vi "TDMS Read Example.vi"() -> ()   [LabVIEW 2016, in "LVtoITX.lvclass"]
uses:
  LVtoITX.lvclass
panel:
  in  "Read Type":enum16{"1 read", "N reads"}(ring)
  out "load time (ms)":u32
  out "Data 2":dbl[][](array[numeric]) format="%#_6p"
  in  "Waves":u16[](array[ring])
  in  "Load Multiple Waves":bool
  in  "Load Wave":bool
  in  "Load Wavenames":bool
  in  "TDMS File path":path
  in  "Stop":bool
  out "Data":dbl[](array[numeric]) format="%#_6p"
  in  "Wave":u16(ring)
  # "^^^^^^^^^^\nPush to populate the ring controls below"
  # "1 read: open file once and get all waves. Choose waves from dictionary after loading\n\nN read: open file for each wave"
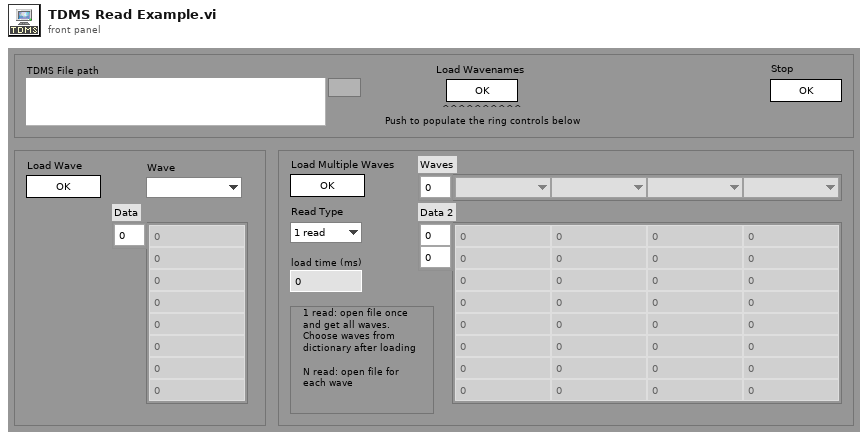
[diagram p1: front panel]
types:
  T1 = enum32{"Invalid", "Standard", "Closed", "Hidden", "Minimized", "Maximized"}
  T2 = enum32{"invalid app kind", "Development System", "Run Time System", "Student Edition", "Embedded LabVIEW", "Evaluation", "Custom"}
  T3 = cluster{"Core":cluster{"Current VI Reference":refnum<vi>, "Close Panel on Exit?":bool}, "TDMS File path":path}
  T4 = cluster{"Current VI Reference":refnum<vi>, "Close Panel on Exit?":bool}
  T5 = typedef "LVtoITX.lvclass/Dictionary--cluster.ctl" = cluster{"key":string, "value":variant}
  T6 = typedef "Dictionary Object RefNum__ogtk.ctl" = refnum<k1>
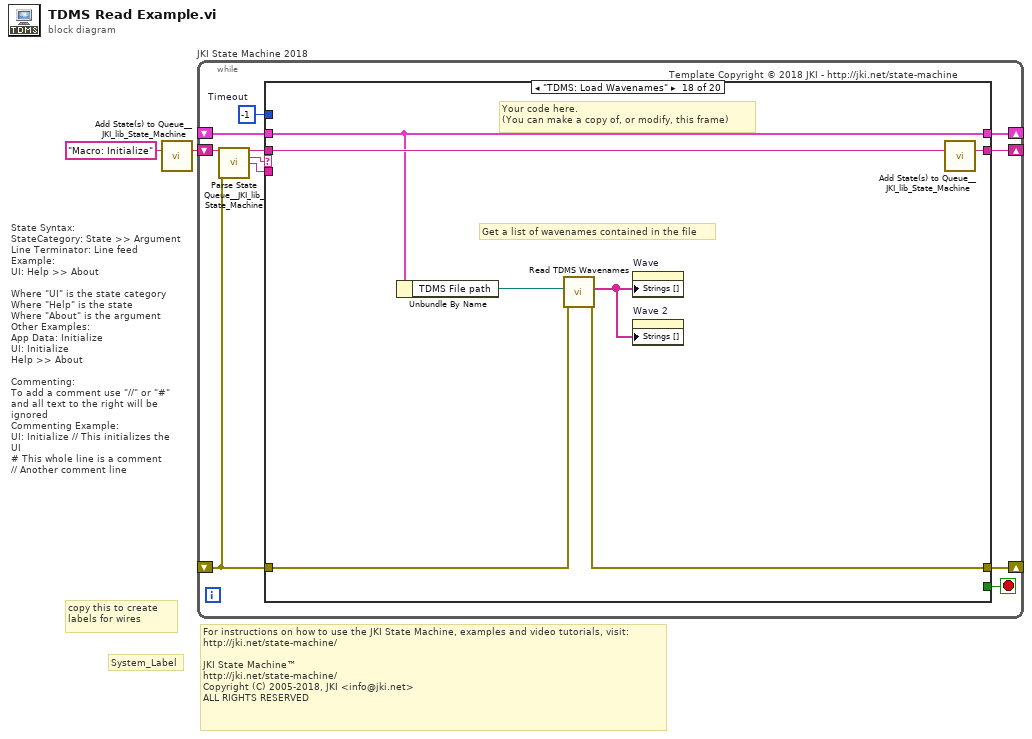
[diagram p0: block diagram]
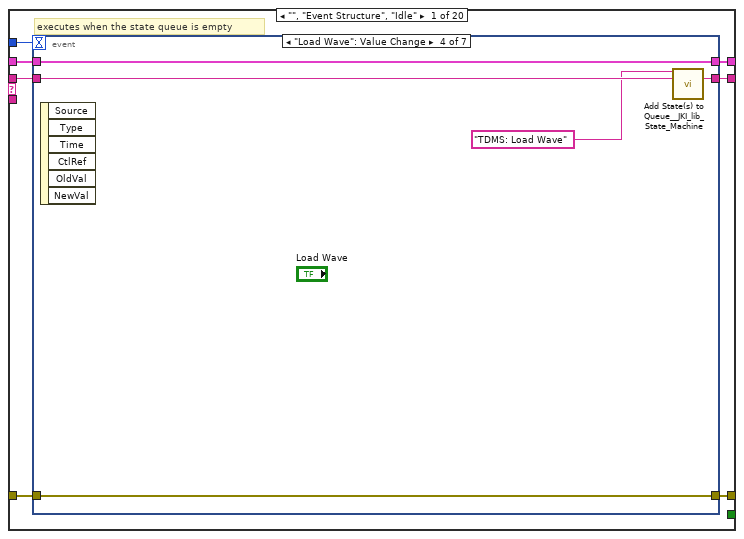
[diagram p2: hidden frame]
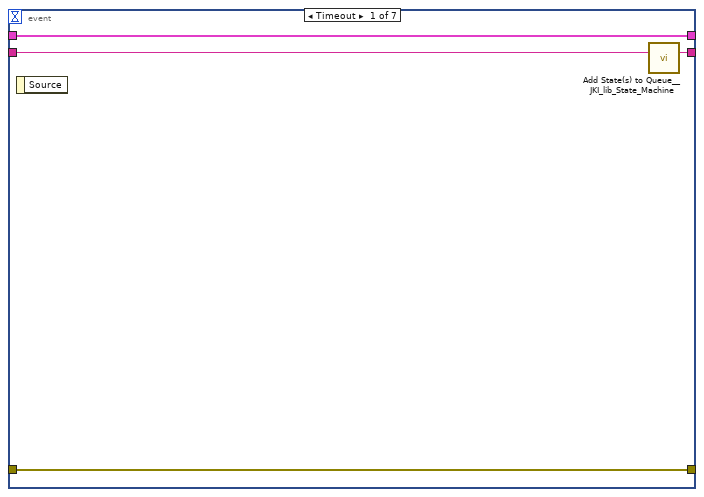
[diagram p3: hidden frame]
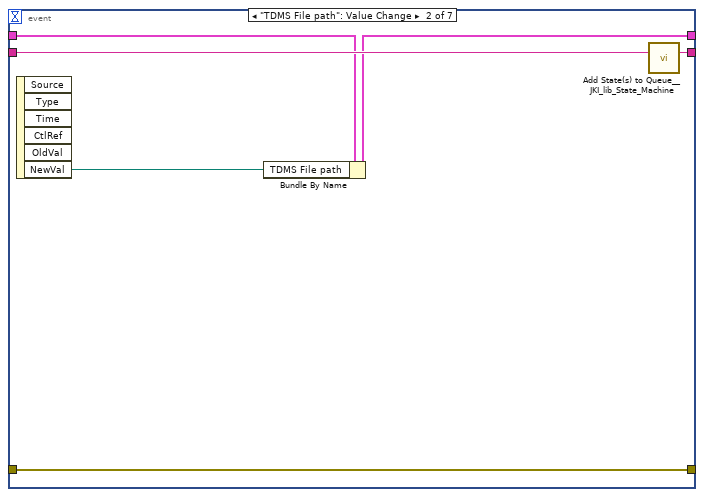
[diagram p4: hidden frame]
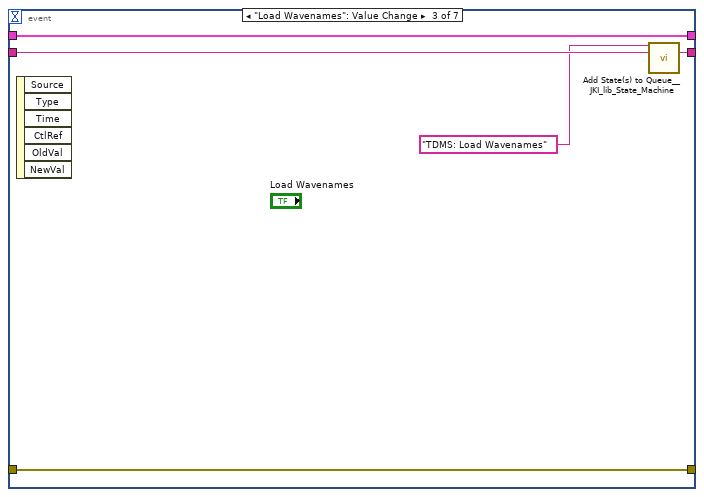
[diagram p5: hidden frame]
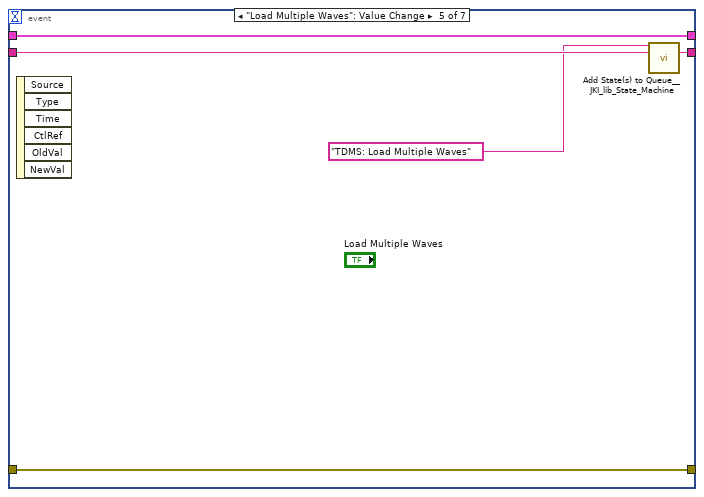
[diagram p6: hidden frame]
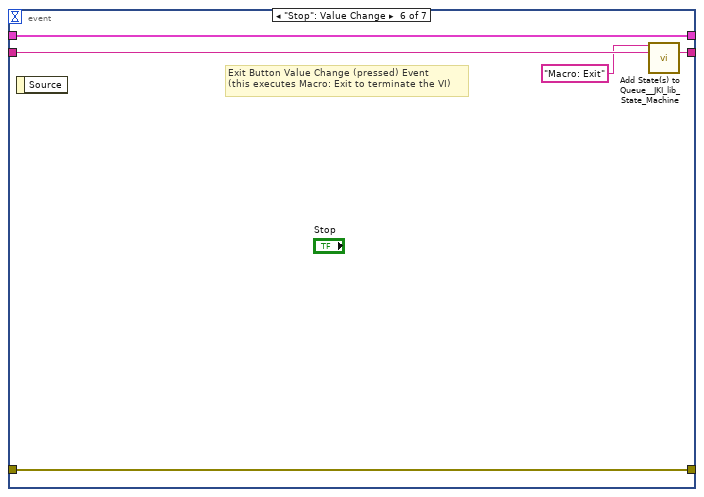
[diagram p7: hidden frame]
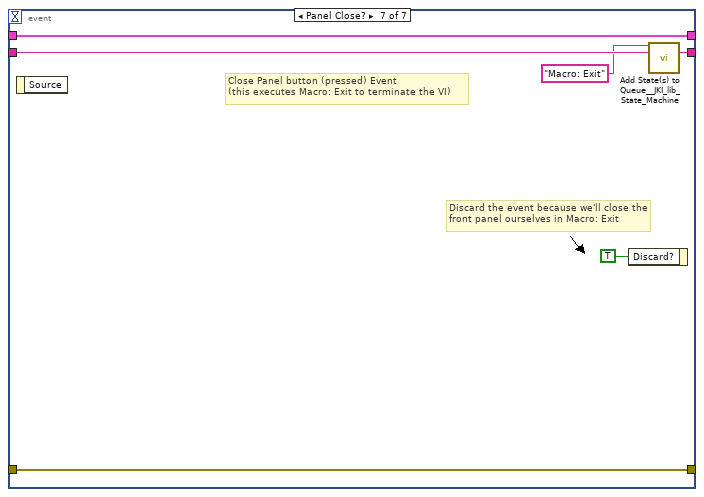
[diagram p8: hidden frame]
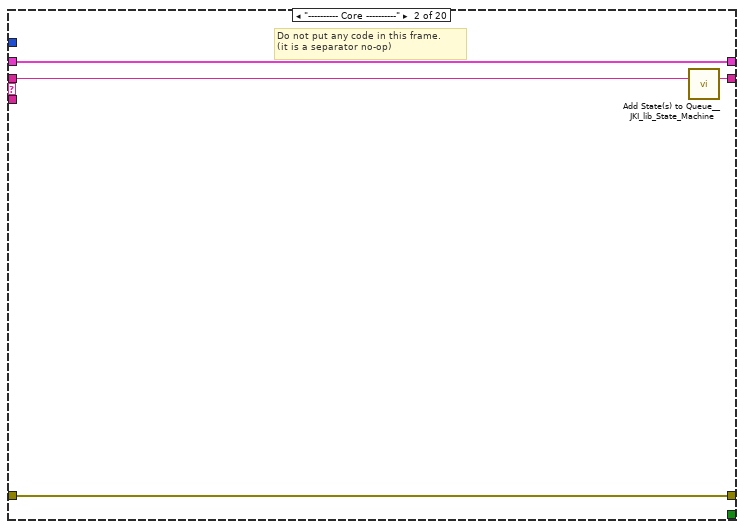
[diagram p9: hidden frame]
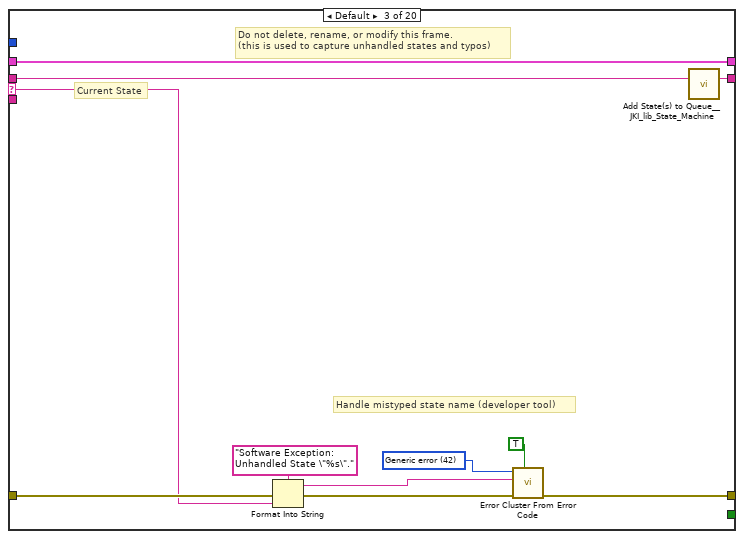
[diagram p10: hidden frame]
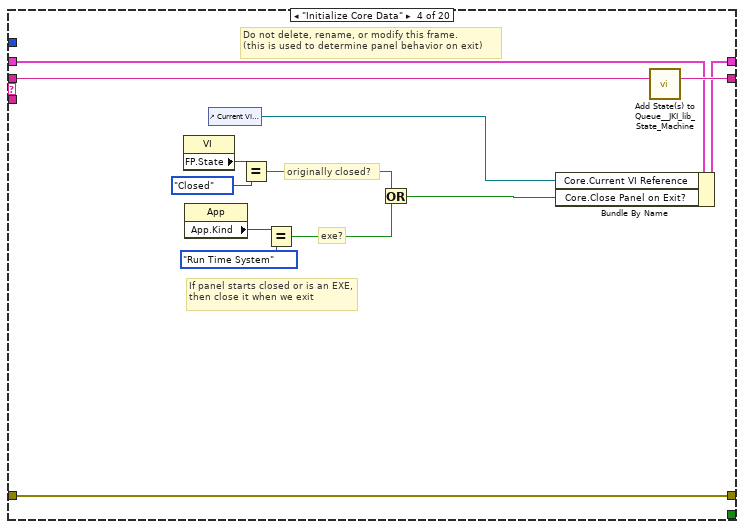
[diagram p11: hidden frame]
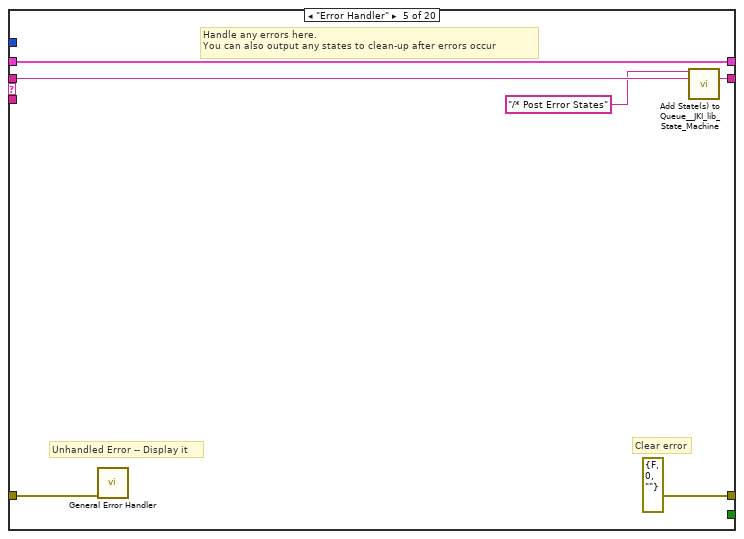
[diagram p12: hidden frame]
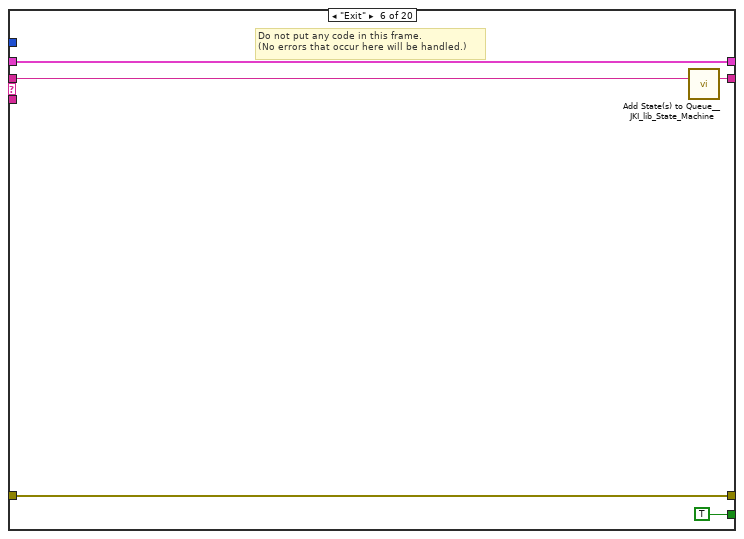
[diagram p13: hidden frame]
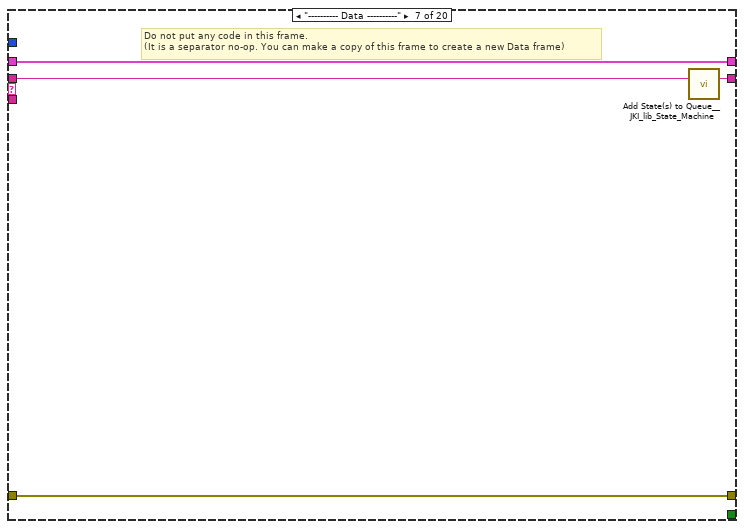
[diagram p14: hidden frame]
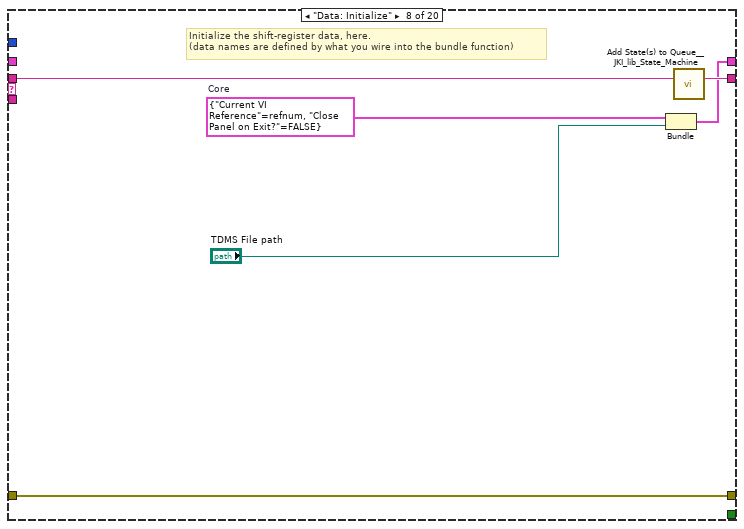
[diagram p15: hidden frame]
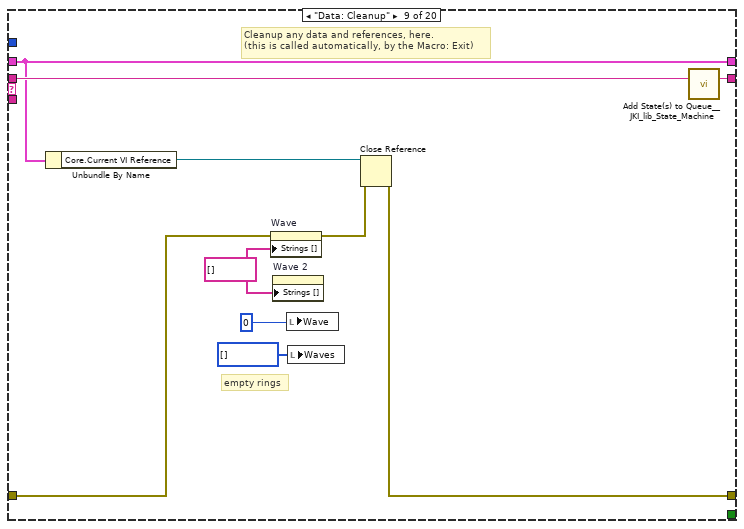
[diagram p16: hidden frame]
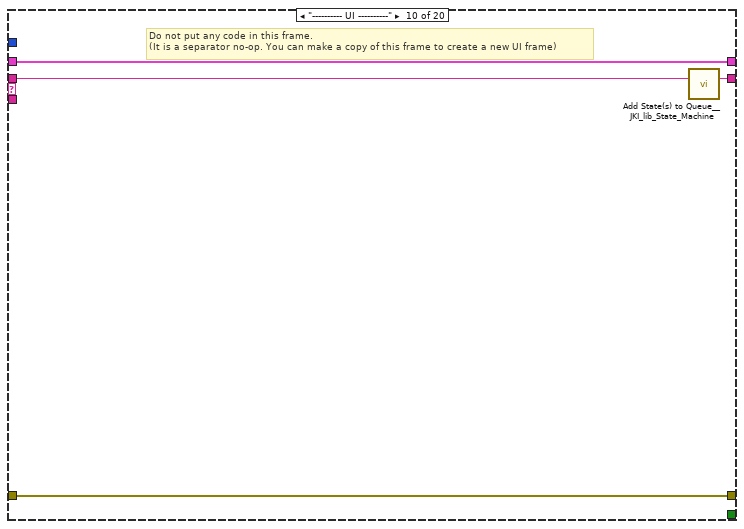
[diagram p17: hidden frame]
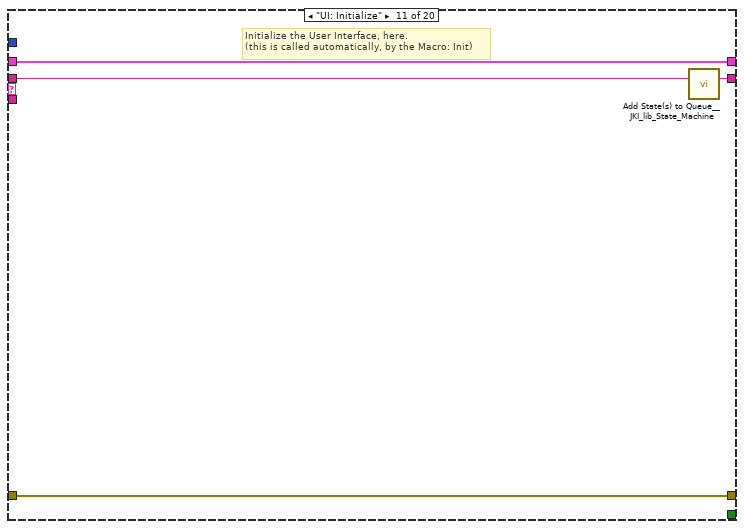
[diagram p18: hidden frame]
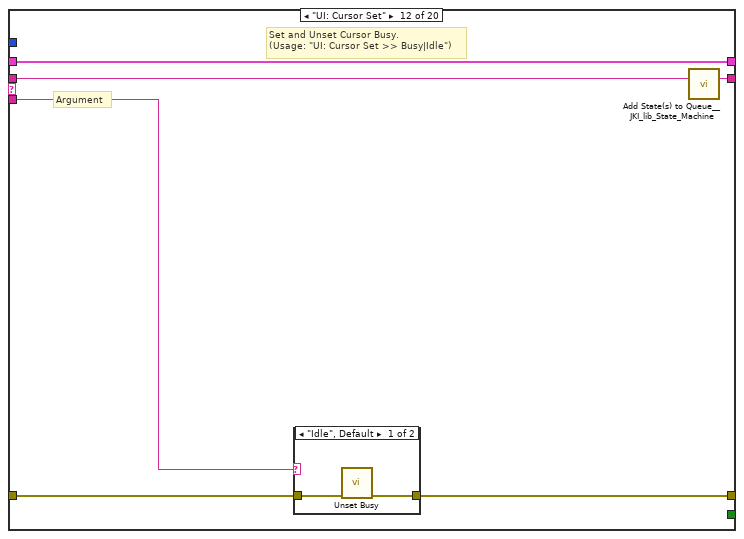
[diagram p19: hidden frame]
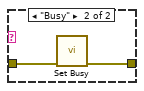
[diagram p20: hidden frame]
diagram:
  # "For instructions on how to use the JKI State Machine, examples and video tutorials, visit:\nhttp://jki.net/state-machine/\n\nJKI State Machine™\nhttp://jki.net/state-machine/\nCopyright (C) 2005-2018, JKI <info@jki.net>\nALL RIGHTS RESERVED"
  # "State Syntax:\nStateCategory: State >> Argument\nLine Terminator: Line feed\nExample:\nUI: Help >> About\n\nWhere \"UI\" is the state category\nWhere \"Help\" is the state\nWhere \"About\" is the argument\nOther Examples:\nApp Data: Initialize\nUI: Initialize\nHelp >> About\n\nCommenting:\nTo add a comment use \"//\" or \"#\" and all text to the right will be ignored\nCommenting Example:\nUI: Initialize // This initializes the UI\n# This whole line is a comment\n// Another comment line"
  # "copy this to create labels for wires"
  # "System_Label"
  n1 = call <vilib>:"Add State(s) to Queue__JKI_lib_State_Machine.vi"("State(s) in (\"\")"="Macro: Initialize") -> ("States Out"=w2:string)  [unwired: 14 in]
  n2 = while "JKI State Machine 2018" {
    shift-right: [w6] -> _
    shift-left: _ -> [w5]
    shift-right: [w9] -> _
    shift-left: _ -> [w3]
    shift-right: [w8] -> _
    shift-left: w2 -> [w10]
    stop <- w7 stop-if-true
    w4 = -1  # Timeout
    # "Template Copyright © 2018 JKI - http://jki.net/state-machine"
    n3 = call <vilib>:"Parse State Queue__JKI_lib_State_Machine.vi"("State Queue"=w10, "Error In (no error)"=w3) -> ("Remaining States"=w12:string, "Current State"=w13:string, "Arguments"=w11:string)  [unwired: 11 in]
    n4 = case shown="\"TDMS: Load Wavenames\"" w13 {
      selector: w13 -> [_ _ w61 _ _ _ _ _ _ _ _ _ _ _ _ _ _ _ _ _]
      tunnel: w12 -> [w20 w60 w65 w84 w90 w95 w99 w105 w115 w119 w123 w129 w140 w209 w214 w224 w228 w235 w245 w261]
      tunnel: w11 -> [_ _ _ _ _ _ _ _ _ _ _ w124 w134 _ _ _ _ _ _ _]
      tunnel: w5 -> [w18 w57 w63 w77 w87 w93 w96 _ w111 w116 w121 w127 w136 w206 w211 w221 w225 w230 w237 w259]
      tunnel: [w17 w58 w67 w81 errorcluster {"status"=FALSE, "code"=0, "source"=""} ("error out") w92 w97 w102 w112 w117 w120 w125 w137 w207 w212 w222 w226 w232 w240 w253] -> w9
      tunnel: w3 -> [w16 w58 w66 w81 w86 w92 w97 w102 w110 w117 w120 w126 w138 w207 w212 w222 w226 w233 w241 w254]
      tunnel: [w19 w59 w64 w83 w89 w94 w98 w104 w114 w118 w122 w128 w139 w208 w213 w223 w227 w234 w244 w260] -> w8
      tunnel: [_ _ _ _ _ TRUE _ _ _ _ _ _ _ _ _ _ _ _ _ _] -> w7
      tunnel: [w15 w57 w63 w82 w87 w93 w96 w103 w111 w116 w121 w127 w136 w206 w211 w221 w225 w230 w237 w259] -> w6
      tunnel: w4 -> [w14 _ _ _ _ _ _ _ _ _ _ _ _ _ _ _ _ _ _ _]
      frame "", "Event Structure", "Idle" {
        # "executes when the state queue is empty"
        n5 = event shown="[3] \"Load Wave\": Value Change" {
          selector: _ -> [_ _ _ _ _ _ _]
          dyn-events: _ -> [_ _ _ _ _ _ _]
          timeout: w14 -> [_ _ _ _ _ _ _]
          tunnel: w20 -> [w24 w30 w35 w40 w45 w50 w56]
          tunnel: [w23 w29 w34 w39 w44 w49 w55] -> w19
          tunnel: w18 -> [w21 w26 w32 w37 w42 w47 w53]
          tunnel: [w22 w28 w33 w38 w43 w48 w54] -> w17
          tunnel: w16 -> [w22 w28 w33 w38 w43 w48 w54]
          tunnel: [w21 w25 w32 w37 w42 w47 w53] -> w15
          event Timeout {
            n6 = event-data() -> ()  [unwired: 1 in, 1 out]
            n7 = call <vilib>:"Add State(s) to Queue__JKI_lib_State_Machine.vi"("State(s) in (\"\")"=w24) -> ("States Out"=w23:string)  [unwired: 14 in]
          }
          event "TDMS File path": Value Change {
            n8 = event-data() -> ("NewVal"=w27:path)  [unwired: 1 in, 5 out]
            n9 = Bundle By Name(cluster=w26, "TDMS File path"=w27) -> (w25:T3)
            n10 = call <vilib>:"Add State(s) to Queue__JKI_lib_State_Machine.vi"("State(s) in (\"\")"=w30) -> ("States Out"=w29:string)  [unwired: 14 in]
          }
          event "Load Wavenames": Value Change {
            n11 = event-data() -> ()  [unwired: 1 in, 6 out]
            n12 = call <vilib>:"Add State(s) to Queue__JKI_lib_State_Machine.vi"("State(s) in Front (\"\")"="TDMS: Load Wavenames" ("State(s) in Front (\"\")"), "State(s) in (\"\")"=w35) -> ("States Out"=w34:string)  [unwired: 13 in]
          }
          event "Load Wave": Value Change {
            n13 = event-data() -> ()  [unwired: 1 in, 6 out]
            n14 = call <vilib>:"Add State(s) to Queue__JKI_lib_State_Machine.vi"("State(s) in Front (\"\")"="TDMS: Load Wave" ("State(s) in Front (\"\")"), "State(s) in (\"\")"=w40) -> ("States Out"=w39:string)  [unwired: 13 in]
          }
          event "Load Multiple Waves": Value Change {
            n15 = event-data() -> ()  [unwired: 1 in, 6 out]
            n16 = call <vilib>:"Add State(s) to Queue__JKI_lib_State_Machine.vi"("State(s) in Front (\"\")"="TDMS: Load Multiple Waves" ("State(s) in Front (\"\")"), "State(s) in (\"\")"=w45) -> ("States Out"=w44:string)  [unwired: 13 in]
          }
          event "Stop": Value Change {
            # "Exit Button Value Change (pressed) Event\n(this executes Macro: Exit to terminate the VI)"
            n17 = event-data() -> ()  [unwired: 1 in, 1 out]
            n18 = call <vilib>:"Add State(s) to Queue__JKI_lib_State_Machine.vi"("State(s) in Front (\"\")"="Macro: Exit", "State(s) in (\"\")"=w50) -> ("States Out"=w49:string)  [unwired: 13 in]
          }
          event Panel Close? {
            # "Discard the event because we'll close the front panel ourselves in Macro: Exit"
            # "Close Panel button (pressed) Event\n(this executes Macro: Exit to terminate the VI)"
            n19 = event-data() -> ()  [unwired: 1 in, 1 out]
            n20 = event-data("Discard?"=TRUE) -> ()  [unwired: 1 in, 1 out]
            n21 = call <vilib>:"Add State(s) to Queue__JKI_lib_State_Machine.vi"("State(s) in Front (\"\")"="Macro: Exit", "State(s) in (\"\")"=w56) -> ("States Out"=w55:string)  [unwired: 13 in]
          }
        }
      }
      frame "---------- Core ----------" {
        # "Do not put any code in this frame.\n(it is a separator no-op)"
        n22 = call <vilib>:"Add State(s) to Queue__JKI_lib_State_Machine.vi"("State(s) in (\"\")"=w60) -> ("States Out"=w59:string)  [unwired: 14 in]
      }
      frame Default {
        w70 = 42 items=["No error", "Argument error", "Memory is full", "Out of zone", "End of file", "File already open", "Generic file I/O error", "File not found", "File permission error", "Disk is full", "Duplicate path", "Too many files open", "System feature not enabled", "Resource file not found", "Cannot add resource", "Resource not found", "Image not found", "Image memory error", "Pen does not exist", "Config type invalid", "Config token not found", "Config parse error", "Config memory error", "Bad external code format", "Bad external code offset", "External code not present", "Null window", "Destroy window error", "Null menu", "Print aborted", "Bad print record", "Print driver error", "Windows error during printing", "Memory error during printing", "Print dialog error", "Generic print error", "Invalid device refnum", "Device not found", "Device parameter error", "Device unit error", "Cannot open device", "Device call aborted", "Generic error", "Cancelled by user", "Object ID too low", "Object ID too high", "Object not in heap", "Unknown heap", "Unknown object (invalid DefProc)", "Unknown object (DefProc not in table)", "Message out of range", "Invalid (null) method", "Unknown message", "Manager call not supported", "Bad address", "Network operation in progress", "Network operation timed out", "Connection is busy", "Network attribute not supported", "Network error", "Address in use", "System out of memory", "Connection aborted", "Connection refused", "Not connected", "Already connected", "Connection closed", "Initialization error (interapplication manager)", "Bad occurrence", "Wait on unbound occurrence handler", "Occurrence queue overflow", "Datalog type conflict", "Unused", "Unrecognized type (interapplication manager)", "Memory corrupt", "Failed to make temporary DLL", "Old CIN version", "Drag socket not found", "Failed to load drop-object", "Failed to register OLE object", "Failed to release OLE object", "Format specifier type mismatch", "Unknown format specifier", "Too few format specifiers", "Too many format specifiers", "Scan failed", "Newer CIN version", "Error converting to variant", "Runtime menu error", "Password tampered", "Variant attribute not found", "Incompatible variant data type", "Event data is not available", "Event Store is not present", "Occurrence is not found", "Event Queue is not created", "Event info is not available", "Refnum passed is NULL", "Error retrieving Class GUID", "Error retrieving CoClass GUID", "Error retrieving TypeLib GUID.", "Bad built application magic bytes.", "Specific driver is different from the specific driver associated with the Logical Name.", "There is no session opened to the class driver.", "Max Error", "MAX - Error with config objects", "MAX - Error loading configuration", "MAX - Group not supported"]
        # "Current State"
        # "Do not delete, rename, or modify this frame.\n(this is used to capture unhandled states and typos)"
        # "Handle mistyped state name (developer tool)"
        n23 = Format Into String(format string="Software Exception: Unhandled State \"%s\"." ("message"), error in=w66, w61) -> (resulting string=w69:string, error out=w68:errorcluster)  [unwired: 1 in]
        n24 = call <vilib>:"Error Cluster From Error Code.vi"("show call chain? (False)"=TRUE, "error in (no error)"=w68, "error message (\"\")"=w69, "error code (0)"=w70) -> ("error out"=w67:errorcluster)  [unwired: 5 in]
        n25 = call <vilib>:"Add State(s) to Queue__JKI_lib_State_Machine.vi"("State(s) in (\"\")"=w65) -> ("States Out"=w64:string)  [unwired: 14 in]
      }
      frame "Initialize Core Data" {
        # "Do not delete, rename, or modify this frame.\n(this is used to determine panel behavior on exit)"
        # "originally closed?"
        # "exe?"
        # "If panel starts closed or is an EXE, then close it when we exit"
        n26 = property class="VI"() -> ("FP.State"=w74:T1)  [unwired: 2 in, 2 out]
        n27 = property class="App"() -> ("App.Kind"=w80:T2)  [unwired: 2 in, 2 out]
        n28 = control-ref of="Current VI Reference"() -> (w75:refnum<vi>)
        n29 = Equal?(x=w74, y=T1."Closed" ("Front Panel Window:State")) -> (x = y?=w72:bool)
        n30 = Equal?(x=w80, y=T2."Run Time System" ("Application:Kind")) -> (x = y?=w78:bool)
        n31 = Or(x=w72, y=w78) -> (x .or. y?=w76:bool)
        n32 = Bundle By Name(cluster=w77, "Core.Current VI Reference"=w75, "Core.Close Panel on Exit?"=w76) -> (w82:T3)
        n33 = call <vilib>:"Add State(s) to Queue__JKI_lib_State_Machine.vi"("State(s) in (\"\")"=w84) -> ("States Out"=w83:string)  [unwired: 14 in]
      }
      frame "Error Handler" {
        # "Unhandled Error -- Display it"
        # "Handle any errors here.\nYou can also output any states to clean-up after errors occur"
        # "Clear error"
        n34 = call <vilib>:"General Error Handler.vi"("error in (no error)"=w86) -> ()  [unwired: 10 in, 5 out]
        n35 = call <vilib>:"Add State(s) to Queue__JKI_lib_State_Machine.vi"("State(s) in Front (\"\")"="/* Post Error States", "State(s) in (\"\")"=w90) -> ("States Out"=w89:string)  [unwired: 13 in]
      }
      frame "Exit" {
        # "Do not put any code in this frame.\n(No errors that occur here will be handled.)"
        n36 = call <vilib>:"Add State(s) to Queue__JKI_lib_State_Machine.vi"("State(s) in (\"\")"=w95) -> ("States Out"=w94:string)  [unwired: 14 in]
      }
      frame "---------- Data ----------" {
        # "Do not put any code in this frame.\n(It is a separator no-op. You can make a copy of this frame to create a new Data frame)"
        n37 = call <vilib>:"Add State(s) to Queue__JKI_lib_State_Machine.vi"("State(s) in (\"\")"=w99) -> ("States Out"=w98:string)  [unwired: 14 in]
      }
      frame "Data: Initialize" {
        w101 = T4 {"Current VI Reference"=refnum, "Close Panel on Exit?"=FALSE}  # Core
        # "Initialize the shift-register data, here.\n(data names are defined by what you wire into the bundle function)"
        n38 = Bundle("Core"=w101, "TDMS File path"="TDMS File path") -> (w103:T3)  [unwired: 1 in]
        n39 = call <vilib>:"Add State(s) to Queue__JKI_lib_State_Machine.vi"("State(s) in (\"\")"=w105) -> ("States Out"=w104:string)  [unwired: 14 in]
      }
      frame "Data: Cleanup" {
        w106 = u16[] [] items=[""] ("Waves")
        w107 = string[] [] ("Strings []")
        # "empty rings"
        # "Cleanup any data and references, here.\n(this is called automatically, by the Macro: Exit)"
        n40 = Unbundle By Name(w111) -> ("Core.Current VI Reference"=w113:refnum<vi>)
        n41 = property on="Wave" class="Ring (strict)"(error in=w110, "Strings []"=w107) -> (error out=w109:errorcluster)  [unwired: 1 in, 1 out]
        n42 = property on="Wave 2" class="Ring (strict)"("Strings []"=w107) -> ()  [unwired: 2 in, 2 out]
        n43 = local write "Wave"(0) -> ()
        n44 = local write "Waves"(w106) -> ()
        n45 = Close Reference(reference=w113, error in (no error)=w109) -> (error out=w112:errorcluster)
        n46 = call <vilib>:"Add State(s) to Queue__JKI_lib_State_Machine.vi"("State(s) in (\"\")"=w115) -> ("States Out"=w114:string)  [unwired: 14 in]
      }
      frame "---------- UI ----------" {
        # "Do not put any code in this frame.\n(It is a separator no-op. You can make a copy of this frame to create a new UI frame)"
        n47 = call <vilib>:"Add State(s) to Queue__JKI_lib_State_Machine.vi"("State(s) in (\"\")"=w119) -> ("States Out"=w118:string)  [unwired: 14 in]
      }
      frame "UI: Initialize" {
        # "Initialize the User Interface, here.\n(this is called automatically, by the Macro: Init)"
        n48 = call <vilib>:"Add State(s) to Queue__JKI_lib_State_Machine.vi"("State(s) in (\"\")"=w123) -> ("States Out"=w122:string)  [unwired: 14 in]
      }
      frame "UI: Cursor Set" {
        # "Argument"
        # "Set and Unset Cursor Busy.\n(Usage: \"UI: Cursor Set >> Busy|Idle\")"
        n49 = case shown="\"Idle\", Default" w124 {
          tunnel: w126 -> [w131 w133]
          tunnel: [w130 w132] -> w125
          frame "Idle", Default {
            n50 = call <vilib>:"Unset Busy.vi"("error in (no error)"=w131) -> ("error out"=w130:errorcluster)  [unwired: 10 in]
          }
          frame "Busy" {
            n51 = call <vilib>:"Set Busy.vi"("error in (no error)"=w133) -> ("error out"=w132:errorcluster)  [unwired: 9 in, 1 out]
          }
        }
        n52 = call <vilib>:"Add State(s) to Queue__JKI_lib_State_Machine.vi"("State(s) in (\"\")"=w129) -> ("States Out"=w128:string)  [unwired: 14 in]
      }
      frame "UI: Front Panel State" {
        # "Argument"
        # "Set Front Panel Open or Closed\n(Usage: \"UI: Front Panel State >> Open|Close\")"
        n53 = Unbundle By Name(w136) -> ("Core.Current VI Reference"=w135:refnum<vi>)
        n54 = case shown="\"Minimize\", \"Minimized\"" w134 {
          tunnel: w138 -> [w146 w161 w172 w185 w198]
          tunnel: [w148 w162 w174 w187 w200] -> w137
          tunnel: w135 -> [w147 w159 w173 w186 w199]
          frame "Open", "Standard", Default {
            w141 = T1."Standard" ("State")
            n55 = property class="VI"(reference=w147, error in=w146) -> (reference out=w144:refnum<vi>, error out=w145:errorcluster, "FP.State"=w143:T1)
            n56 = Not Equal?(x=w143, y=w141) -> (x != y?=w142:bool)
            n57 = case shown="True" w142 {
              tunnel: [w152 w154] -> w148
              tunnel: w145 -> [w151 w154]
              tunnel: w144 -> [w150 _]
              tunnel: w141 -> [w149 _]
              frame True {
                n58 = invoke class="VI" method="FP.Open"(reference=w150, error in=w151, "Activate"=TRUE, "State"=w149) -> (error out=w152:errorcluster)  [unwired: 1 in, 4 out]
              }
              frame False {
              }
            }
          }
          frame "Close", "Closed" {
            n59 = property class="VI"(reference=w159, error in=w161) -> (reference out=w158:refnum<vi>, error out=w160:errorcluster, "FP.State"=w156:T1)
            n60 = Not Equal?(x=w156, y=T1."Closed" ("Front Panel Window:State")) -> (x != y?=w155:bool)
            n61 = case shown="True" w155 {
              tunnel: [w163 w166] -> w162
              tunnel: w160 -> [w163 w165]
              tunnel: w158 -> [_ w164]
              frame False {
              }
              frame True {
                n62 = invoke class="VI" method="FP.Close"(reference=w164, error in=w165) -> (error out=w166:errorcluster)  [unwired: 1 in, 2 out]
              }
            }
          }
          frame "Hidden", "Hide" {
            w167 = T1."Hidden" ("State")
            n63 = property class="VI"(reference=w173, error in=w172) -> (reference out=w170:refnum<vi>, error out=w171:errorcluster, "FP.State"=w169:T1)
            n64 = Not Equal?(x=w169, y=w167) -> (x != y?=w168:bool)
            n65 = case shown="True" w168 {
              tunnel: [w178 w179] -> w174
              tunnel: w171 -> [w177 w179]
              tunnel: w170 -> [w176 _]
              tunnel: w167 -> [w175 _]
              frame True {
                n66 = invoke class="VI" method="FP.Open"(reference=w176, error in=w177, "State"=w175) -> (error out=w178:errorcluster)  [unwired: 2 in, 4 out]
              }
              frame False {
              }
            }
          }
          frame "Minimize", "Minimized" {
            w180 = T1."Minimized" ("State")
            n67 = property class="VI"(reference=w186, error in=w185) -> (reference out=w183:refnum<vi>, error out=w184:errorcluster, "FP.State"=w182:T1)
            n68 = Not Equal?(x=w182, y=w180) -> (x != y?=w181:bool)
            n69 = case shown="True" w181 {
              tunnel: [w191 w192] -> w187
              tunnel: w184 -> [w190 w192]
              tunnel: w183 -> [w189 _]
              tunnel: w180 -> [w188 _]
              frame True {
                n70 = invoke class="VI" method="FP.Open"(reference=w189, error in=w190, "State"=w188) -> (error out=w191:errorcluster)  [unwired: 2 in, 4 out]
              }
              frame False {
              }
            }
          }
          frame "Maximize", "Maximized" {
            w193 = T1."Maximized" ("State")
            n71 = property class="VI"(reference=w199, error in=w198) -> (reference out=w196:refnum<vi>, error out=w197:errorcluster, "FP.State"=w195:T1)
            n72 = Not Equal?(x=w195, y=w193) -> (x != y?=w194:bool)
            n73 = case shown="True" w194 {
              tunnel: [w204 w205] -> w200
              tunnel: w197 -> [w203 w205]
              tunnel: w196 -> [w202 _]
              tunnel: w193 -> [w201 _]
              frame True {
                n74 = invoke class="VI" method="FP.Open"(reference=w202, error in=w203, "State"=w201) -> (error out=w204:errorcluster)  [unwired: 2 in, 4 out]
              }
              frame False {
              }
            }
          }
        }
        n75 = call <vilib>:"Add State(s) to Queue__JKI_lib_State_Machine.vi"("State(s) in (\"\")"=w140) -> ("States Out"=w139:string)  [unwired: 14 in]
      }
      frame "---------- Macro ----------" {
        # "Do not put any code in this frame.\n(It is a separator no-op. You can make a copy of this frame to create a new Macro frame)"
        n76 = call <vilib>:"Add State(s) to Queue__JKI_lib_State_Machine.vi"("State(s) in (\"\")"=w209) -> ("States Out"=w208:string)  [unwired: 14 in]
      }
      frame "Macro: Initialize" {
        w210 = "Data: Initialize\nInitialize Core Data\nUI: Initialize\nUI: Front Panel State >> Open"  # Data: Initialize Initialize Core Data UI: Initialize UI: Front Panel State >> Open
        # "Initialization Macro\n(This is called once, when the VI starts)"
        n77 = call <vilib>:"Add State(s) to Queue__JKI_lib_State_Machine.vi"("State(s) in Front (\"\")"=w210, "State(s) in (\"\")"=w214) -> ("States Out"=w213:string)  [unwired: 13 in]
      }
      frame "Macro: Exit" {
        # "Exit Macro\n(This is called once, when the VI exits)"
        n78 = Unbundle By Name(w221) -> ("Core.Close Panel on Exit?"=w220:bool)
        n79 = Select(t="UI: Front Panel State >> Close", s=w220, f="") -> (s? t:f=w217:string)
        n80 = call <vilib>:"Add State(s) to Queue__JKI_lib_State_Machine.vi"("State(s) in (\"\")"=w217, "State(s) at Back (\"\")"="Data: Cleanup\nExit") -> ("States Out"=w215:string)  [unwired: 13 in]
        n81 = call <vilib>:"Add State(s) to Queue__JKI_lib_State_Machine.vi"("State(s) in Front (\"\")"=w215, "State(s) in (\"\")"=w224) -> ("States Out"=w223:string)  [unwired: 13 in]
      }
      frame "---------- TDMS ----------" {
        # "Template Separator\n(You can make a copy of, or modify, this frame)"
        n82 = call <vilib>:"Add State(s) to Queue__JKI_lib_State_Machine.vi"("State(s) in (\"\")"=w228) -> ("States Out"=w227:string)  [unwired: 14 in]
      }
      frame "TDMS: Load Wavenames" {
        # "Get a list of wavenames contained in the file"
        # "Your code here.\n(You can make a copy of, or modify, this frame)"
        n83 = Unbundle By Name(w230) -> ("TDMS File path"=w229:path)
        n84 = call "Read TDMS Wavenames.vi"("error in (no error)"=w233, "path"=w229) -> ("error out"=w232:errorcluster, "Wavenames"=w231:string[])  [unwired: 7 in, 1 out]
        n85 = property on="Wave" class="Ring (strict)"("Strings []"=w231) -> ()  [unwired: 2 in, 2 out]
        n86 = property on="Wave 2" class="Ring (strict)"("Strings []"=w231) -> ()  [unwired: 2 in, 2 out]
        n87 = call <vilib>:"Add State(s) to Queue__JKI_lib_State_Machine.vi"("State(s) in (\"\")"=w235) -> ("States Out"=w234:string)  [unwired: 14 in]
      }
      frame "TDMS: Load Wave" {
        # "Your code here.\n(You can make a copy of, or modify, this frame)"
        n88 = Unbundle By Name(w237) -> ("TDMS File path"=w236:path)
        n89 = property on="Wave" class="Ring (strict)"() -> ("Strings []"=w243:string[])  [unwired: 2 in, 2 out]
        n90 = Index Array(array=w243, index="Wave") -> (element=w242:string)
        n91 = call "Read TDMS Wave.vi"("error in (no error)"=w241, "channel name(s) in"=w242, "path"=w236) -> ("error out"=w240:errorcluster, "data"=→"Data":dbl[])  [unwired: 6 in, 1 out]
        n92 = call <vilib>:"Add State(s) to Queue__JKI_lib_State_Machine.vi"("State(s) in (\"\")"=w245) -> ("States Out"=w244:string)  [unwired: 14 in]
      }
      frame "TDMS: Load Multiple Waves" {
        # "Template Separator\n(You can make a copy of, or modify, this frame)"
        n93 = Unbundle By Name(w259) -> ("TDMS File path"=w258:path)
        n94 = property on="Wave 2" class="Ring (strict)"() -> ("Strings []"=w256:string[])  [unwired: 2 in, 2 out]
        n95 = call <userlib>:"Tick Count (ms)__ogtk.vi"("error in (no error)"=w254) -> ("error out"=w251:errorcluster, "millisecond timer value"=w250:u32)  [unwired: 9 in]
        n96 = case shown="\"1 read\", Default" "Read Type" {
          tunnel: w258 -> [w272 w289]
          tunnel: "Waves" -> [w269 w287]
          tunnel: w256 -> [w268 w286]
          tunnel: [w266 w285] -> w255
          tunnel: [w264 w284] -> w252
          tunnel: w251 -> [w263 w288]
          frame "1 read", Default {
            n97 = call "Read TDMS.vi"("error in (no error)"=w263, "path"=w272) -> ("error out"=w267:errorcluster, "Data (Dictionary)"=w271:T5[])  [unwired: 3 in, 5 out]
            n98 = call <userlib>:"Dictionary Create__ogtk.vi"("error in (no error)"=w267, "initial dictionary (empty)"=w271) -> ("error out"=w270:errorcluster, "dictionary out"=w262:T6)  [unwired: 8 in]
            n99 = for {
              tunnel: w262 -> [w283]
              tunnel: w270 -> [w282]
              tunnel: w269 -> [w281] mode=indexing
              tunnel: w268 -> [w280]
              tunnel: [w273] -> w266 mode=indexing
              tunnel: [w275] -> w265
              tunnel: [w274] -> _
              n100 = Index Array(array=w280, index=w281) -> (element=w279:string)
              n101 = call <userlib>:"Dictionary Get Value__ogtk.vi"("error in"=w282, "key"=w279, "dictionary"=w283) -> ("error out"=w278:errorcluster, "value"=w276:variant, "dictionary out"=w274:T6)  [unwired: 5 in, 1 out]
              n102 = Variant To Data(error in=w278, type=dbl[] [] ("array type (2D Dbl)"), Variant=w276) -> (data=w273:dbl[], error out=w275:errorcluster)
            }
            n103 = call <userlib>:"Dictionary Destroy__ogtk.vi"("error in (no error)"=w265, "dictionary"=w262) -> ("error out"=w264:errorcluster)  [unwired: 9 in]
          }
          frame "N reads" {
            n104 = for {
              tunnel: w289 -> [w296]
              tunnel: w288 -> [w295]
              tunnel: w287 -> [w294] mode=indexing
              tunnel: w286 -> [w293]
              tunnel: [w291] -> w285 mode=indexing
              tunnel: [w290] -> w284
              n105 = Index Array(array=w293, index=w294) -> (element=w292:string)
              n106 = call "Read TDMS Wave.vi"("error in (no error)"=w295, "channel name(s) in"=w292, "path"=w296) -> ("error out"=w290:errorcluster, "data"=w291:dbl[])  [unwired: 6 in, 1 out]
            }
          }
        }
        n107 = Transpose 2D Array(2D array=w255) -> (transposed array=→"Data 2":dbl[][])
        n108 = call <userlib>:"Tick Count (ms)__ogtk.vi"("error in (no error)"=w252) -> ("error out"=w253:errorcluster, "millisecond timer value"=w249:u32)  [unwired: 9 in]
        n109 = Subtract(x=w249, y=w250) -> (x-y=→"load time (ms)":u32)
        n110 = call <vilib>:"Add State(s) to Queue__JKI_lib_State_Machine.vi"("State(s) in (\"\")"=w261) -> ("States Out"=w260:string)  [unwired: 14 in]
      }
    }
  }
